vi "LVClass_HasoField Get Strehl From PSF.vi"(0 "HasoField in":refnum<class "HasoField.lvclass">, 1 "Oversample":bool, 5 "Haso configuration file":path, 7 "experimental_psf":refnum<class "SurfaceFloat.lvclass">, 9 "theoretical_psf":refnum<class "SurfaceFloat.lvclass">, 11 "error in (no error)":errorcluster) -> (4 "HasoField out":refnum<class "HasoField.lvclass">, 6 "Strehl Ratio":dbl, 15 "error out":errorcluster)   [LabVIEW 2020, in "HasoField.lvclass"]
uses:
  HasoField.lvclass
  SurfaceFloat.lvclass
  HasoField.lvclass/HasoField.ctl
  LVClasse_SurfaceFloat Read SurfaceFloat.vi
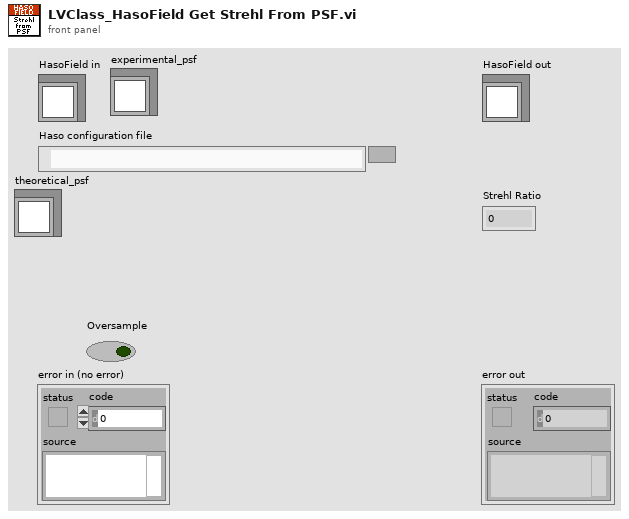
[diagram p1: front panel]
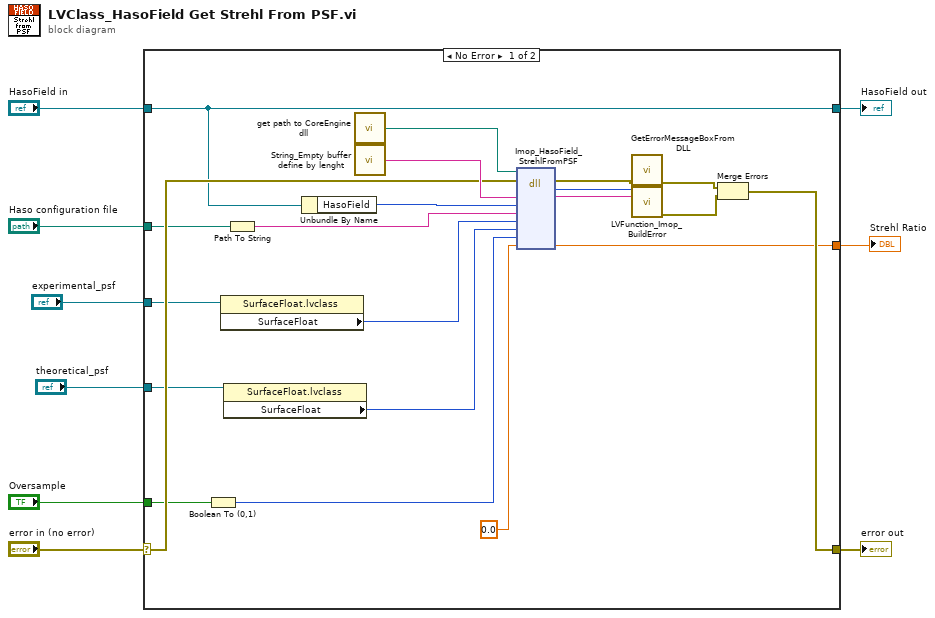
[diagram p0: block diagram]
diagram:
  n1 = case shown="No Error" "error in (no error)" {
    selector: "error in (no error)" -> [w23 w32]
    tunnel: [w22 w32] -> w8
    tunnel: [w21 w31] -> w6
    tunnel: "HasoField in" -> [w21 w31]
    tunnel: "Haso configuration file" -> [w19 _]
    tunnel: "Oversample" -> [w17 _]
    tunnel: [w14 _] -> w3
    tunnel: "experimental_psf" -> [w13 _]
    tunnel: "theoretical_psf" -> [w11 _]
    frame No Error {
      n2 = Boolean To (0,1)(Boolean=w17) -> (0, 1=w16:i16)
      n3 = property class="SurfaceFloat.lvclass"(reference=w13) -> ("SurfaceFloat"=w12:i32)  [unwired: 1 in, 2 out]
      n4 = property class="SurfaceFloat.lvclass"(reference=w11) -> ("SurfaceFloat"=w10:i32)  [unwired: 1 in, 2 out]
      n5 = Path To String(path=w19) -> (string=w18:string)
      n6 = Unbundle By Name(w21) -> ("HasoField"=w20:i32)
      n7 = call "get path to CoreEngine dll.vi"() -> ("path to c_interface_vc100.dll"=w30:path)  [unwired: 12 in, 3 out]
      n8 = call "String_Empty buffer define by lenght.vi"() -> ("Empty buffer"=w29:string)  [unwired: 1 in]
      n9 = dll-call lib="D:/FLE/0.Code/CoreEngine4_Suite/LV2011_interface/DLLs/c_interface_vc100.dll" fn="Imop_HasoField_StrehlFromPSF"(path in=w30, error in=w23, "message"=w29, "hasofield"=w20, "haso_config_file_path"=w18, "Experimental PSF"=w12, "Theorical PSF"=w10, "Oversample"=w16, "Strehl ratio"=sgl 0.0) -> (error out=w28:errorcluster, "return type"=w25:i32, "message"=w24:string, "Strehl ratio"=w14:sgl)  [unwired: 6 in, 1 out]
      n10 = call "GetErrorMessageBoxFromDLL.vi"("error IN"=w28) -> ("error OUT"=w27:errorcluster)  [unwired: 10 in]
      n11 = call "LVFunction_Imop_BuildError.vi"("code"=w25, "String to Prepend to source (\"\")"=w24) -> ("error out"=w26:errorcluster)  [unwired: 13 in]
      n12 = Merge Errors(w27, w26) -> (w22:errorcluster)
    }
    frame Error {
    }
  }
  "error out" <- w8
  "HasoField out" <- w6
  "Strehl Ratio" <- w3
